vi "READ - Multiple Wave Files.vi"(0 "reference in":refnum<class "WaveFile.lvclass">, 5 "error in (no error)":errorcluster, 7 "READ - Multiple Files":path[](array[path])) -> (14 "reference out":refnum<class "WaveFile.lvclass">, 19 "error out":errorcluster)   [LabVIEW 2022 SP3, in "WaveFile.lvclass"]
uses:
  WaveFile.lvclass
  W:/projects/archives/23 Charette AI Group/SPWB/API/Generic Utilities_class/Generic Utilities.lvclass
  API/GSwFormDSP_class/GSwFormDSP.lvclass
  API/Generic Utilities_class/Generic Utilities.lvclass
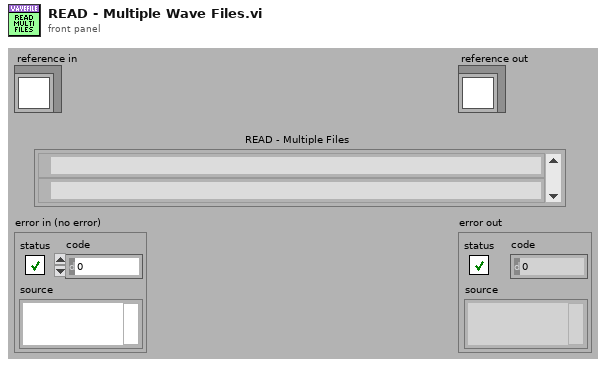
[diagram p1: front panel]
types:
  T1 = typedef "Generic Utilities.lvclass/GUI Parameters.ctl" = cluster{"Application Name":string, "GUI VI Ref":refnum<vi>, "Close Panel?":bool, "Message Window ref":refnum<vi>, "Version #":string}
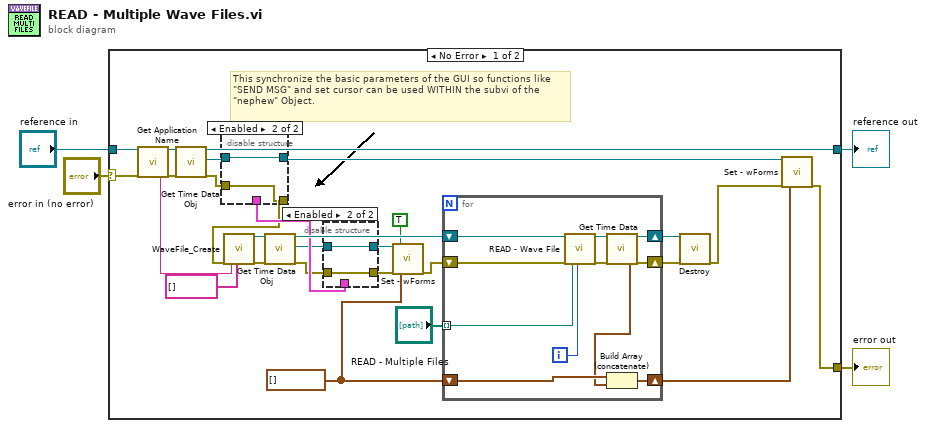
[diagram p0: block diagram]
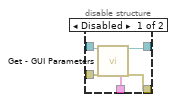
[diagram p2: hidden frame]
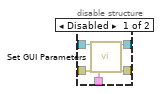
[diagram p3: hidden frame]
diagram:
  n1 = case shown="No Error" "error in (no error)" {
    selector: "error in (no error)" -> [w11 w59]
    tunnel: [w25 w59] -> w3
    tunnel: [w32 w58] -> w1
    tunnel: "reference in" -> [w12 w58]
    frame No Error {
      w22 = waveform(dbl)[] []
      # "This synchronize the basic parameters of the GUI so functions like \"SEND MSG\" and set cursor can be used WITHIN the subvi of the \"nephew\" Object."
      n2 = call "Get Application Name.vi"("reference in"=w12, "error in (no error)"=w11) -> ("Application Name"=w31:string, "reference out"=w13:refnum<class "WaveFile.lvclass">, "error out"=w10:errorcluster)  [unwired: 15 in]
      n3 = call "Get Time Data Obj.vi"("reference in"=w13, "error in (no error)"=w10) -> ("reference out"=w32:refnum<class "WaveFile.lvclass">, "Time data ref"=w9:refnum<class "GSwFormDSP.lvclass">, "error out"=w6:errorcluster)  [unwired: 15 in]
      n4 = disable-structure shown="Enabled" {
        disable-tunnel: [w37 _] -> w20
        disable-tunnel: w9 -> [w36 w39]
        disable-tunnel: [w35 w39] -> w8
        disable-tunnel: w6 -> [w34 w38]
        disable-tunnel: [w33 w38] -> w5
        frame Disabled {
          n5 = call "Get - GUI Parameters.vi"("reference in"=w36, "error in (no error)"=w34) -> ("GUI Parameters"=w37:T1, "reference out"=w35:refnum<class "GSwFormDSP.lvclass">, "error out"=w33:errorcluster)  [unwired: 15 in]
        }
        frame Enabled {
        }
      }
      n6 = call "WaveFile_Create.vi"("error in (no error)"=w5, "Application Name"=w31, "State Queue"=string[] []) -> ("reference out"=w19:refnum<class "WaveFile.lvclass">, "error out"=w18:errorcluster)  [unwired: 15 in]
      n7 = call "Get Time Data Obj.vi"("reference in"=w19, "error in (no error)"=w18) -> ("reference out"=w24:refnum<class "WaveFile.lvclass">, "Time data ref"=w17:refnum<class "GSwFormDSP.lvclass">, "error out"=w15:errorcluster)  [unwired: 15 in]
      n8 = disable-structure shown="Enabled" {
        disable-tunnel: w20 -> [w44 _]
        disable-tunnel: w17 -> [w43 w46]
        disable-tunnel: [w42 w46] -> w16
        disable-tunnel: w15 -> [w41 w45]
        disable-tunnel: [w40 w45] -> w14
        frame Disabled {
          n9 = call "Set GUI Parameters.vi"("reference in"=w43, "error in (no error)"=w41, "GUI Parameters"=w44) -> ("reference out"=w42:refnum<class "GSwFormDSP.lvclass">, "error out"=w40:errorcluster)  [unwired: 15 in]
        }
        frame Enabled {
        }
      }
      n10 = call "Set - wForms.vi"("reference in"=w16, "error in (no error)"=w14, "Init wForms"=TRUE, "wForms"=w22) -> ("error out"=w23:errorcluster)  [unwired: 14 in, 1 out]
      n11 = for {
        shift-right: [w53] -> w26
        shift-left: w23 -> [w47]
        shift-right: [w54] -> w27
        shift-left: w24 -> [w57]
        tunnel: "READ - Multiple Files" -> [w49] mode=indexing
        shift-right: [w52] -> w28
        shift-left: w22 -> [w51]
        i -> [w48]
        n12 = call "READ - Wave File.vi"("reference in"=w57, "error in (no error)"=w47, "Wave File Path - READ"=w49, "Channel Offset (0 => ignore)"=w48) -> ("reference out"=w56:refnum<class "WaveFile.lvclass">, "error out"=w55:errorcluster)  [unwired: 14 in]
        n13 = call "Get Time Data.vi"("reference in"=w56, "error in (no error)"=w55) -> ("wForms"=w50:waveform(dbl)[], "reference out"=w54:refnum<class "WaveFile.lvclass">, "error out"=w53:errorcluster)  [unwired: 14 in, 1 out]
        n14 = Build Array (concatenate)(w51, w50) -> (w52:waveform(dbl)[])
      }
      n15 = call-dynamic "Destroy.vi"("reference in"=w27, "error in (no error)"=w26) -> ("error out"=w7:errorcluster)  [unwired: 16 in, 1 out]
      n16 = call "Set - wForms.vi"("reference in"=w8, "error in (no error)"=w7, "wForms"=w28) -> ("error out"=w25:errorcluster)  [unwired: 15 in, 1 out]
    }
    frame Error {
    }
  }
  "error out" <- w3
  "reference out" <- w1
